vi "BestY for any element.vi"(7 "Element Position":dbl[](array[numeric]), 8 "error in (no error)":errorcluster, 9 "Enemys(T)\nAllys(F)":bool=TRUE, 10 "Game":refnum<class "Game.lvclass">, 11 "Utilities in":refnum<class "Utilities.lvclass">) -> (0 "error out":errorcluster, 2 "Goal Gap Normalizado(%do gol aberta)":dbl, 3 "Utilities out":refnum<class "Utilities.lvclass">)   [LabVIEW 2018, in "Utilities.lvclass"]
uses:
  Utilities.lvclass
  segment.ctl
  Game_class/Game.lvclass
  Game_class/Game.lvclass/Game.ctl
  Team_class/Team.lvclass/Team.ctl
  Object_class/Object.lvclass/Object.ctl
  Object_class/Read x.vi
  Object_class/Read y.vi
  <vilib>/Analysis/baseanly.llb/Real Dot Product.vi
  Game_class/Read FieldRef.vi
  Game_class/Read EnemyRef.vi
  Game_class/Read AllyRef.vi
  Team_class/Read RobotRef.vi
  Ally_class/Ally.lvclass
  Enemy_class/Enemy.lvclass
  Robot_class/Robot.lvclass
  Field_class/Field.lvclass
  <vilib>/Analysis/NI_AALBase.lvlib
panel:
  out "Vetor de gaps \ncorreto":T1[](array[typedef])
  out "Eclipse":bool
  out "Gap Coord":dbl[](array[numeric])
  out "Goal Gap":dbl
  out "Vetor de gaps":T1[](array[typedef])
  in  "Maior intervalo(T)\nMaior angulo(F)":bool
  in  "eclipse angle eps":dbl=0.035 format="%#_13g"
  out "Best y(for kick target)":dbl
  out "pilha output (merged)":T1[](array[typedef])
  out "Vetor de segmentos ordenado":T1[](array[typedef])
  out "Vetor de segmentos (sombras)":T1[](array[typedef])
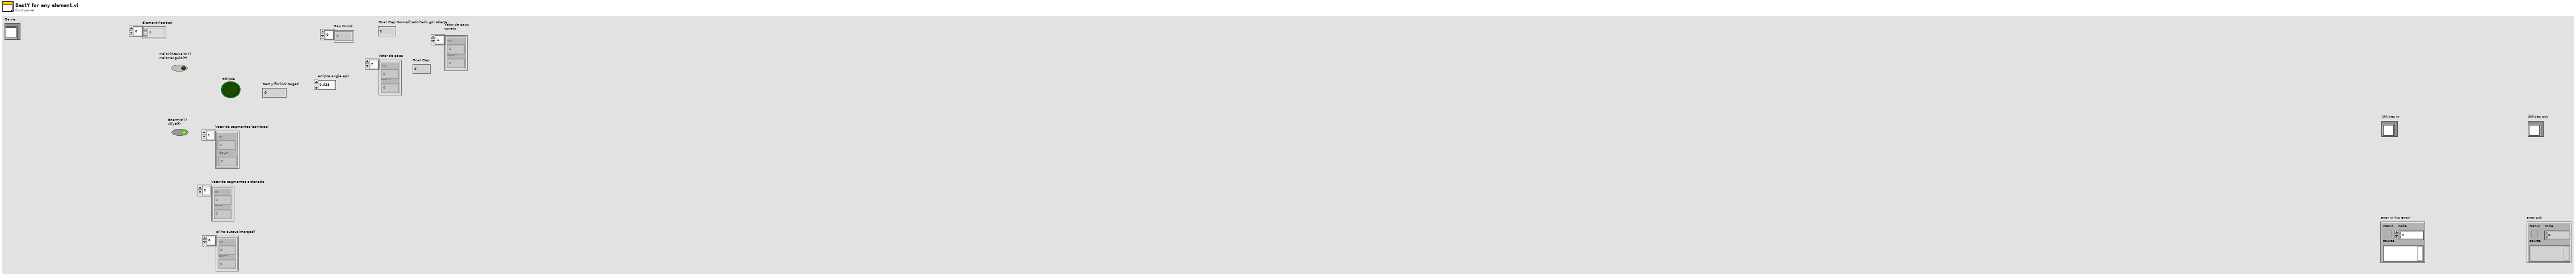
[diagram p1: front panel]
types:
  T1 = typedef "Utilities.lvclass/segment.ctl" = cluster{"up":dbl, "down":dbl}
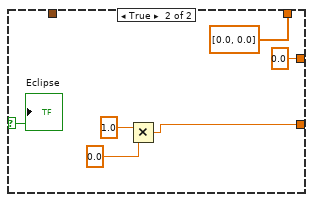
[diagram p4: hidden frame]
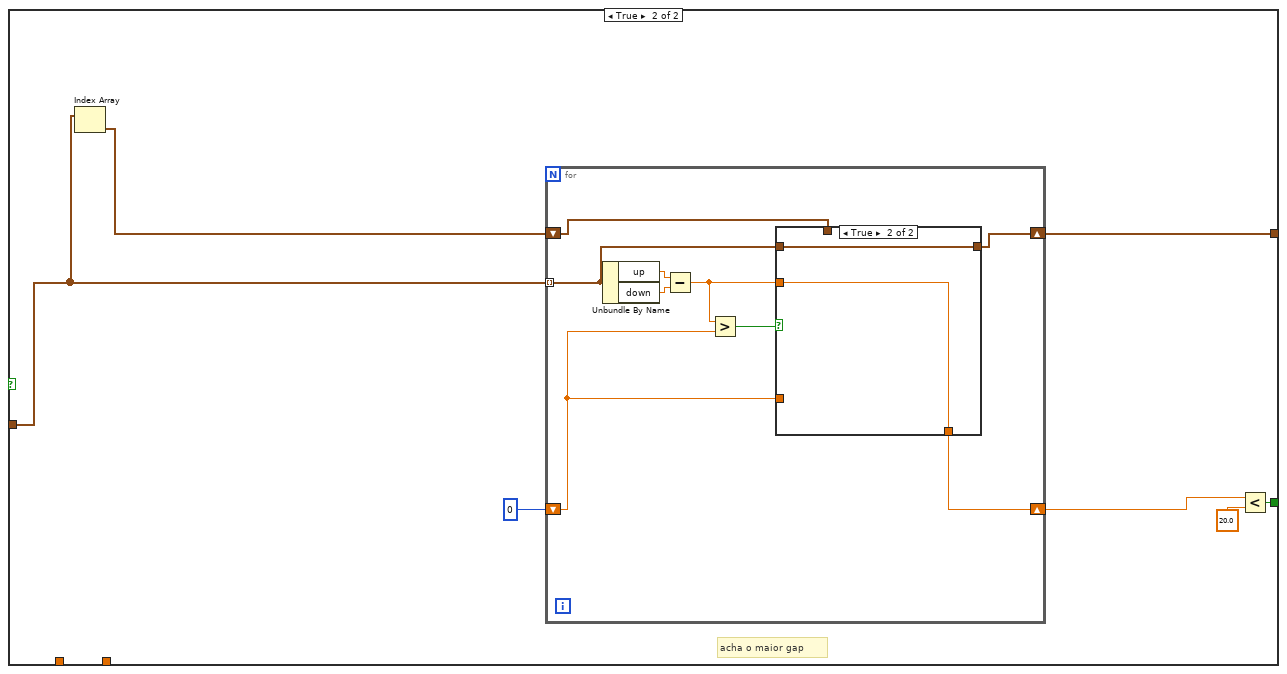
[diagram p6: hidden frame]
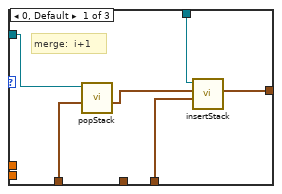
[diagram p8: hidden frame]
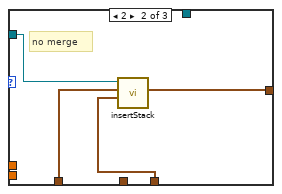
[diagram p9: hidden frame]
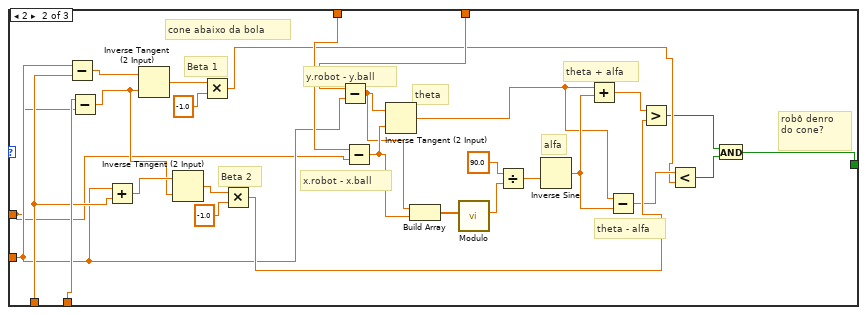
[diagram p11: hidden frame]
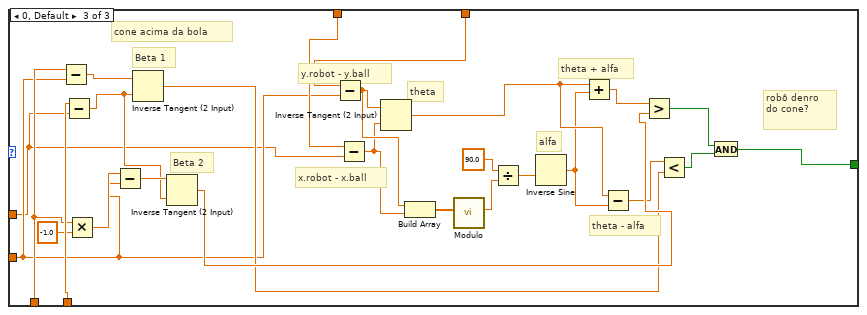
[diagram p12: hidden frame]
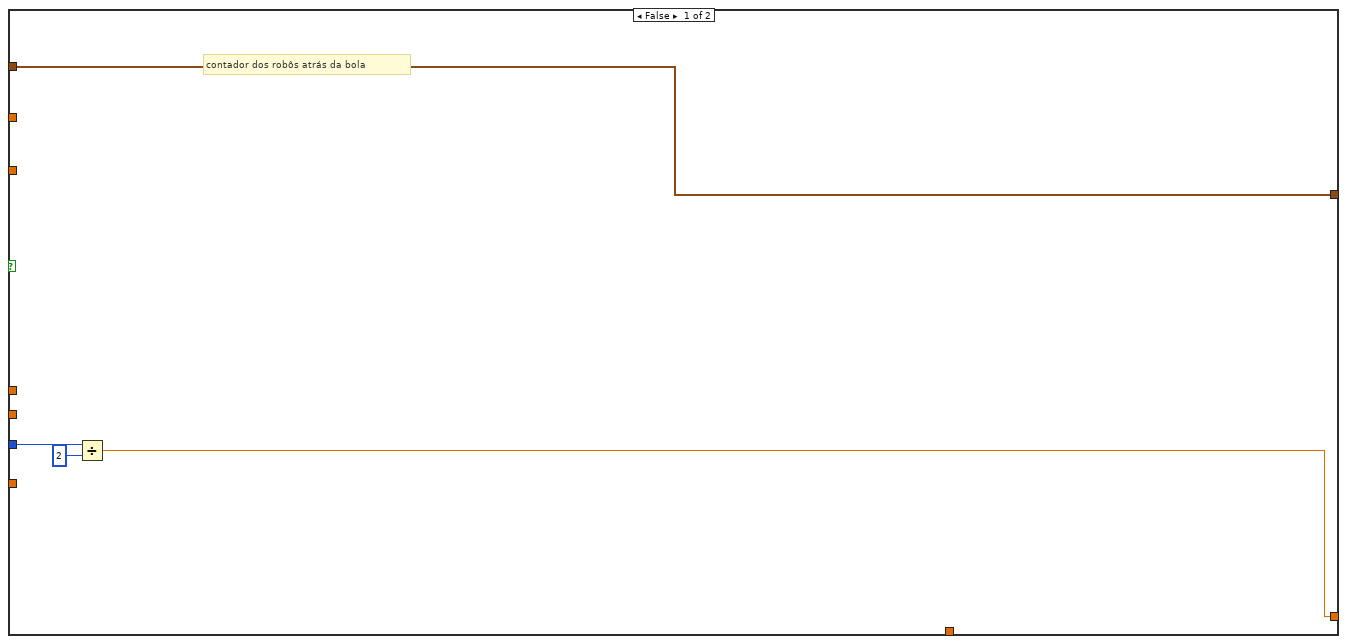
[diagram p13: hidden frame]
diagram:
  n1 = case shown="No Error" "error in (no error)" {
    selector: "error in (no error)" -> [w51 w398]
    tunnel: [w51 w398] -> w5
    tunnel: [w7 w397] -> w3
    tunnel: "Utilities in" -> [w7 w397]
    tunnel: "Game" -> [w9 _]
    tunnel: "Enemys(T)\nAllys(F)" -> [w8 _]
    frame No Error {
      # "default T"
      # "Default FALSE"
      # "goal_width/2"
      # "field_length/2"
      # "balls"
      # "vetor de gaps"
      # "upper"
      # "Wire the error cluster across even in the \"No Error\"\ncase so that warnings get propagated."
      n2 = property class="Game"(reference=w9) -> ("FieldRef"=w16:refnum<class "Field.lvclass">, "EnemyRef"=w13:refnum<class "Enemy.lvclass">, "AllyRef"=w12:refnum<class "Ally.lvclass">)  [unwired: 1 in, 2 out]
      n3 = property class="Enemy"(reference=w13) -> ("RobotRef"=w10:refnum<class "Robot.lvclass">[])  [unwired: 1 in, 2 out]
      n4 = property class="Ally"(reference=w12) -> ("RobotRef"=w11:refnum<class "Robot.lvclass">[])  [unwired: 1 in, 2 out]
      n5 = property class="Field"(reference=w16) -> ("field_length"=w15:i32, "field_width"=w14:i32)  [unwired: 1 in, 2 out]
      n6 = Select(t=w10, s=w8, f=w11) -> (s? t:f=w33:refnum<class "Robot.lvclass">[])
      n7 = Divide(x=w14, y=u32 2 ("x")) -> (x/y=w25:dbl)
      n8 = To Double Precision Float(number=w14) -> (double precision float=w17:dbl)
      n9 = for {
        shift-right: [w245] -> w36
        shift-left: T1[] [] -> [w244]
        tunnel: w15 -> [w223]
        tunnel: w25 -> [w225]
        tunnel: w25 -> [w242]
        shift-right: [w241] -> w34
        shift-left: _ -> [_]
        tunnel: w33 -> [w214] mode=indexing
        tunnel: w8 -> [w239]
        tunnel: "Element Position" -> [w217]
        # "y element"
        # "x element"
        # "y.robot"
        # "x.robot"
        # "field_length/2"
        # "goal_width/2"
        # "y element"
        # "x element"
        n10 = property class="Robot"(reference=w214) -> ("x"=w213:dbl, "y"=w212:dbl)  [unwired: 1 in, 2 out]
        n11 = Index Array(array=w217) -> (element #1=w216:dbl, element #2=w215:dbl)  [unwired: 2 in]
        n12 = Multiply(x=w213, y=-1.0) -> (x*y=w238:dbl)
        n13 = Absolute Value(x=w216) -> (abs(x)=w237:dbl)
        n14 = Absolute Value(x=w213) -> (abs(x)=w243:dbl)
        n15 = Select(t=w213, s=w239, f=w238) -> (s? t:f=w220:dbl)
        n16 = Greater?(x=w243, y=w237) -> (0:w218:bool)
        n17 = Multiply(x=w225, y=-1.0) -> (x*y=w229:dbl)
        n18 = Greater?(x=w215, y=w225) -> (0:w228:bool)
        n19 = Less?(x=w215, y=w229) -> (x < y?=w227:bool)
        n20 = Select(t=1, s=w228, f=0) -> (s? t:f=w235:i32)
        n21 = Select(t=0, s=w227, f=1) -> (s? t:f=w236:i32)
        n22 = Add(x=w235, y=w236) -> (x+y=w226:i32)
        n23 = Divide(x=w223, y=2.0) -> (x/y=w222:dbl)
        n24 = case shown="1" w226 {
          tunnel: w225 -> [w248 w274 w322]
          tunnel: w222 -> [w269 w294 w324]
          tunnel: w220 -> [w256 w281 w317]
          tunnel: w212 -> [w255 w282 w318]
          tunnel: [w257 w283 w308] -> w219
          tunnel: w216 -> [w246 w272 w300]
          tunnel: w215 -> [w247 w273 w301]
          frame 1 {
            # "robô denro\ndo cone?"
            # "cone centrado"
            # "theta - alfa"
            # "theta + alfa"
            # "theta"
            # "alfa"
            # "x.robot - x.element"
            # "y.robot - y.element"
            # "Beta 2"
            # "Beta 1"
            n25 = Subtract(x=w248, y=w247) -> (x-y=w270:dbl)
            n26 = Subtract(x=w269, y=w246) -> (x-y=w271:dbl)
            n27 = Add(x=w247, y=w248) -> (x+y=w268:dbl)
            n28 = Inverse Tangent (2 Input)(1:w271, 2:w270) -> (0:w251:dbl)
            n29 = Inverse Tangent (2 Input)(1:w271, 2:w268) -> (0:w267:dbl)
            n30 = Multiply(x=w267, y=-1.0) -> (x*y=w253:dbl)
            n31 = Subtract(x=w255, y=w247) -> (x-y=w258:dbl)
            n32 = Subtract(x=w256, y=w246) -> (x-y=w259:dbl)
            n33 = Inverse Tangent (2 Input)(1:w259, 2:w258) -> (0:w264:dbl)
            n34 = Build Array(w258, w259) -> (w260:dbl[])
            n35 = call "Modulo.vi"("2D vector"=w260) -> ("Modulo"=w261:dbl)  [unwired: 10 in]
            n36 = Divide(x=90.0, y=w261) -> (x/y=w262:dbl)
            n37 = Inverse Sine(1:w262) -> (0:w265:dbl)
            n38 = Add(x=w264, y=w265) -> (x+y=w254:dbl)
            n39 = Subtract(x=w264, y=w265) -> (x-y=w252:dbl)
            n40 = Greater?(x=w254, y=w253) -> (0:w249:bool)
            n41 = Less?(x=w252, y=w251) -> (x < y?=w250:bool)
            n42 = And(x=w249, y=w250) -> (x .and. y?=w257:bool)
          }
          frame 2 {
            # "robô denro\ndo cone?"
            # "cone abaixo da bola"
            # "theta - alfa"
            # "theta + alfa"
            # "theta"
            # "alfa"
            # "x.robot - x.ball"
            # "y.robot - y.ball"
            # "Beta 2"
            # "Beta 1"
            n43 = Subtract(x=w273, y=w274) -> (x-y=w296:dbl)
            n44 = Subtract(x=w294, y=w272) -> (x-y=w295:dbl)
            n45 = Add(x=w273, y=w274) -> (x+y=w297:dbl)
            n46 = Inverse Tangent (2 Input)(1:w295, 2:w296) -> (0:w292:dbl)
            n47 = Inverse Tangent (2 Input)(1:w295, 2:w297) -> (0:w298:dbl)
            n48 = Multiply(x=w292, y=-1.0) -> (x*y=w277:dbl)
            n49 = Multiply(x=w298, y=-1.0) -> (x*y=w279:dbl)
            n50 = Subtract(x=w282, y=w273) -> (x-y=w284:dbl)
            n51 = Subtract(x=w281, y=w272) -> (x-y=w285:dbl)
            n52 = Inverse Tangent (2 Input)(1:w285, 2:w284) -> (0:w290:dbl)
            n53 = Build Array(w284, w285) -> (w286:dbl[])
            n54 = call "Modulo.vi"("2D vector"=w286) -> ("Modulo"=w287:dbl)  [unwired: 10 in]
            n55 = Divide(x=90.0, y=w287) -> (x/y=w288:dbl)
            n56 = Inverse Sine(1:w288) -> (0:w291:dbl)
            n57 = Add(x=w290, y=w291) -> (x+y=w280:dbl)
            n58 = Subtract(x=w290, y=w291) -> (x-y=w278:dbl)
            n59 = Greater?(x=w280, y=w279) -> (0:w275:bool)
            n60 = Less?(x=w278, y=w277) -> (x < y?=w276:bool)
            n61 = And(x=w275, y=w276) -> (x .and. y?=w283:bool)
          }
          frame 0, Default {
            # "robô denro\ndo cone?"
            # "cone acima da bola"
            # "theta - alfa"
            # "theta + alfa"
            # "theta"
            # "alfa"
            # "x.robot - x.ball"
            # "y.robot - y.ball"
            # "Beta 2"
            # "Beta 1"
            n62 = Subtract(x=w322, y=w301) -> (x-y=w325:dbl)
            n63 = Subtract(x=w324, y=w300) -> (x-y=w319:dbl)
            n64 = Multiply(x=w322, y=-1.0) -> (x*y=w321:dbl)
            n65 = Subtract(x=w321, y=w301) -> (x-y=w320:dbl)
            n66 = Inverse Tangent (2 Input)(1:w319, 2:w325) -> (0:w303:dbl)
            n67 = Inverse Tangent (2 Input)(1:w319, 2:w320) -> (0:w306:dbl)
            n68 = Subtract(x=w318, y=w301) -> (x-y=w316:dbl)
            n69 = Subtract(x=w317, y=w300) -> (x-y=w315:dbl)
            n70 = Inverse Tangent (2 Input)(1:w315, 2:w316) -> (0:w310:dbl)
            n71 = Build Array(w316, w315) -> (w314:dbl[])
            n72 = call "Modulo.vi"("2D vector"=w314) -> ("Modulo"=w313:dbl)  [unwired: 10 in]
            n73 = Divide(x=90.0, y=w313) -> (x/y=w312:dbl)
            n74 = Inverse Sine(1:w312) -> (0:w309:dbl)
            n75 = Add(x=w310, y=w309) -> (x+y=w307:dbl)
            n76 = Subtract(x=w310, y=w309) -> (x-y=w304:dbl)
            n77 = Greater?(x=w307, y=w306) -> (0:w305:bool)
            n78 = Less?(x=w304, y=w303) -> (x < y?=w302:bool)
            n79 = And(x=w305, y=w302) -> (x .and. y?=w308:bool)
          }
        }
        n80 = And(x=w218, y=w219) -> (x .and. y?=w221:bool)
        n81 = case shown="True" w221 {
          tunnel: [w329 w336] -> w245
          tunnel: w244 -> [w329 w338]
          tunnel: w223 -> [w328 w343]
          tunnel: w225 -> [_ w342]
          tunnel: w242 -> [_ w335]
          tunnel: [w326 w334] -> w241
          tunnel: w212 -> [_ w333]
          tunnel: w220 -> [_ w332]
          tunnel: w216 -> [_ w330]
          tunnel: w215 -> [_ w331]
          frame False {
            # "contador dos robôs atrás da bola"
            n82 = Divide(x=w328, y=u32 2) -> (x/y=w326:dbl)
          }
          frame True {
            n83 = flat-sequence {
              tunnel: w333 -> [w378]
              tunnel: w343 -> [w374]
              tunnel: w342 -> [w359]
              tunnel: [w349] -> w341
              tunnel: [w348] -> w340
              tunnel: [w360] -> w339
              tunnel: w338 -> [w353]
              tunnel: [w353] -> w337
              tunnel: [w347] -> w334
              tunnel: w332 -> [w346]
              tunnel: w331 -> [w344]
              tunnel: w330 -> [w345]
              tunnel: w341 -> [w382]
              tunnel: w340 -> [w381]
              tunnel: w339 -> [w383]
              tunnel: w337 -> [w384]
              tunnel: [w380] -> w336
              tunnel: w335 -> [w379]
              frame #0 {
                # "theta - alfa"
                # "alfa + theta"
                # "theta"
                # "alfa"
                # "x.robot - x.element"
                # "y.robot - y.element"
                n84 = Divide(x=w374, y=u32 2 ("x")) -> (x/y=w347:dbl)
                n85 = Subtract(x=w346, y=w345) -> (x-y=w357:dbl)
                n86 = Subtract(x=w378, y=w344) -> (x-y=w358:dbl)
                n87 = Multiply(x=w359, y=-1.0) -> (x*y=w365:dbl)
                n88 = Subtract(x=w347, y=w345) -> (x-y=w350:dbl)
                n89 = Inverse Tangent (2 Input)(1:w357, 2:w358) -> (0:w356:dbl)
                n90 = Build Array(w358, w357) -> (w377:dbl[])
                n91 = call "Modulo.vi"("2D vector"=w377) -> ("Modulo"=w375:dbl)  [unwired: 10 in]
                n92 = Divide(x=90.0, y=w375) -> (x/y=w355:dbl)
                n93 = Inverse Sine(1:w355) -> (0:w354:dbl)
                n94 = Subtract(x=w356, y=w354) -> (x-y=w370:dbl)
                n95 = Tangent(1:w370) -> (0:w369:dbl)
                n96 = Add(x=w356, y=w354) -> (x+y=w372:dbl)
                n97 = Tangent(1:w372) -> (0:w371:dbl)
                n98 = Multiply(x=w369, y=w350) -> (x*y=w351:dbl)
                n99 = Multiply(x=w371, y=w350) -> (x*y=w352:dbl)
                n100 = Add(x=w351, y=w344) -> (x+y=w348:dbl)
                n101 = Add(x=w352, y=w344) -> (x+y=w349:dbl)
                n102 = Less?(x=w349, y=w365) -> (x < y?=w364:bool)
                n103 = Less?(x=w348, y=w365) -> (x < y?=w363:bool)
                n104 = Greater?(x=w348, y=w359) -> (0:w367:bool)
                n105 = Greater?(x=w349, y=w359) -> (0:w368:bool)
                n106 = And(x=w368, y=w367) -> (x .and. y?=w362:bool)
                n107 = And(x=w364, y=w363) -> (x .and. y?=w361:bool)
                n108 = Or(x=w362, y=w361) -> (x .or. y?=w360:bool)
              }
              frame #1 {
                # "goal_width/2"
                n109 = case shown="False" w383 {
                  tunnel: [w393 w396] -> w380
                  tunnel: w384 -> [w392 w396]
                  tunnel: w382 -> [w391 _]
                  tunnel: w381 -> [w389 _]
                  tunnel: w379 -> [w388 _]
                  frame False {
                    n110 = Max & Min(x=w391, y=w388) -> (min(x,y)=w390:dbl)  [unwired: 1 out]
                    n111 = Multiply(x=w388, y=-1.0) -> (x*y=w386:dbl)
                    n112 = Max & Min(x=w389, y=w386) -> (max(x,y)=w385:dbl)  [unwired: 1 out]
                    n113 = Bundle(cluster=T1 {"up"=0.0, "down"=0.0} ("segment 2"), "up"=w390, "down"=w385) -> (w394:T1)
                    n114 = Insert Into Array(array=w392, new element=w394) -> (w393:T1[])  [unwired: 1 in]
                  }
                  frame True {
                  }
                }
              }
            }
          }
        }
      }
      "Vetor de segmentos (sombras)" <- w36
      n115 = Sort 1D Array(array=w36) -> (sorted array=w48:T1[])
      "Vetor de segmentos ordenado" <- w48
      n116 = Index Array(array=w48) -> (element=w47:T1)  [unwired: 1 in]
      n117 = call-dynamic "insertStack.vi"("novo elemento"=w47, "pilha input"=T1[] [], "Utilities in"=w7) -> ("pilha output"=w45:T1[])  [unwired: 5 in, 2 out]
      n118 = for {
        shift-right: [w171] -> w44
        shift-left: w45 -> [w173]
        tunnel: w48 -> [w172] mode=indexing
        i -> [w174]
        n119 = case shown="Default" w174 {
          tunnel: w173 -> [w179 w211]
          tunnel: w172 -> [w182 _]
          tunnel: [w180 w211] -> w171
          frame Default {
            w175 = refnum<class "Utilities.lvclass"> refnum ("Utilities in")
            # "pilha"
            # "i+1"
            # "i"
            # "i+1"
            # "i"
            n120 = call-dynamic "topStack.vi"("pilha input"=w179, "Utilities in"=w175) -> ("top"=w181:T1)  [unwired: 7 in, 2 out]
            n121 = Unbundle By Name(w181) -> ("up"=w178:dbl, "down"=w183:dbl)
            n122 = Unbundle By Name(w182) -> ("down"=w177:dbl, "up"=w184:dbl)
            n123 = Greater Or Equal?(x=w177, y=w178) -> (x >= y?=w176:bool)
            n124 = Less?(x=w177, y=w183) -> (x < y?=w186:bool)
            n125 = Select(t=1, s=w176, f=0) -> (s? t:f=w188:i32)
            n126 = Select(t=0, s=w186, f=1) -> (s? t:f=w187:i32)
            n127 = Add(x=w188, y=w187) -> (x+y=w185:i32)
            n128 = case shown="1" w185 {
              tunnel: w184 -> [_ _ w209]
              tunnel: w183 -> [_ _ w208]
              tunnel: w181 -> [_ _ _]
              tunnel: w182 -> [w195 w201 _]
              tunnel: [w198 w200 w204] -> w180
              tunnel: w179 -> [w197 w202 w207]
              tunnel: w175 -> [w194 _ _]
              tunnel: w175 -> [w193 w199 w203]
              frame 0, Default {
                # "merge:  i+1"
                n129 = call-dynamic "popStack.vi"("pilha input"=w197, "Utilities in"=w193) -> ("pilha output"=w196:T1[])  [unwired: 7 in, 2 out]
                n130 = call-dynamic "insertStack.vi"("novo elemento"=w195, "pilha input"=w196, "Utilities in"=w194) -> ("pilha output"=w198:T1[])  [unwired: 5 in, 2 out]
              }
              frame 2 {
                # "no merge"
                n131 = call-dynamic "insertStack.vi"("novo elemento"=w201, "pilha input"=w202, "Utilities in"=w199) -> ("pilha output"=w200:T1[])  [unwired: 5 in, 2 out]
              }
              frame 1 {
                # "merge top i+1 down i"
                n132 = Bundle(cluster=T1 {"up"=0.0, "down"=0.0} ("segment 2"), "up"=w209, "down"=w208) -> (w205:T1)
                n133 = call-dynamic "popStack.vi"("pilha input"=w207, "Utilities in"=w203) -> ("pilha output"=w206:T1[])  [unwired: 7 in, 2 out]
                n134 = call-dynamic "insertStack.vi"("novo elemento"=w205, "pilha input"=w206, "Utilities in"=w203) -> ("pilha output"=w204:T1[])  [unwired: 5 in, 2 out]
              }
            }
          }
          frame 0 {
          }
        }
      }
      "pilha output (merged)" <- w44
      n135 = Reverse 1D Array(array=w44) -> (reversed array=w43:T1[])
      n136 = for {
        tunnel: w43 -> [w170] mode=indexing
        shift-right: [w164] -> w40
        shift-left: T1[] [] -> [w166]
        shift-right: [w165] -> w39
        shift-left: w25 -> [w167]
        n137 = Unbundle By Name(w170) -> ("up"=w163:dbl, "down"=w165:dbl)
        n138 = Bundle(cluster=T1 {"up"=0.0, "down"=0.0} ("segment 2"), "up"=w167, "down"=w163) -> (w169:T1)
        n139 = Insert Into Array(array=w166, new element=w169) -> (w164:T1[])  [unwired: 1 in]
      }
      n140 = Multiply(x=w25, y=-1.0) -> (x*y=w37:dbl)
      n141 = Bundle(cluster=T1 {"up"=0.0, "down"=0.0} ("segment 2"), "up"=w39, "down"=w37) -> (w42:T1)
      n142 = Insert Into Array(array=w40, new element=w42) -> (w26:T1[])  [unwired: 1 in]
      n143 = Array Size(array=w26) -> (size(s)=w28:i32)
      n144 = Decrement(x=w28) -> (x-1=w27:i32)
      n145 = for {
        N: w27 -> [_]
        shift-right: [w70] -> w24
        shift-left: w26 -> [w72]
        i -> [w71]
        n146 = Increment(x=w71) -> (x+1=w80:i32)
        n147 = Index Array(array=w72, index=w71) -> (element=w73:T1)
        n148 = Index Array(array=w72, index=w80) -> (element=w79:T1)
        n149 = Unbundle By Name(w79) -> ("up"=w77:dbl, "down"=w74:dbl)
        n150 = Unbundle By Name(w73) -> ("up"=w75:dbl, "down"=w78:dbl)
        n151 = Equal?(x=w78, y=w77) -> (x = y?=w76:bool)
        n152 = case shown="True" w76 {
          tunnel: w75 -> [_ w90]
          tunnel: w74 -> [_ w89]
          tunnel: w73 -> [_ w88]
          tunnel: w72 -> [w81 w86]
          tunnel: w71 -> [_ w83]
          tunnel: [w81 w82] -> w70
          frame False {
          }
          frame True {
            n153 = Bundle By Name(cluster=w88, "up"=w90, "down"=w89) -> (w84:T1)
            n154 = Delete From Array(array=w86, length=2, index=w83) -> (array with subset deleted=w85:T1[])  [unwired: 1 out]
            n155 = Insert Into Array(array=w85, index=w83, new element=w84) -> (w82:T1[])
          }
        }
      }
      "Vetor de gaps" <- w24
      n156 = for {
        tunnel: w25 -> [w61]
        tunnel: w24 -> [w54] mode=indexing
        shift-right: [w56] -> w21
        shift-left: T1[] [] -> [w55]
        n157 = Unbundle By Name(w54) -> ("up"=w53:dbl, "down"=w52:dbl)
        n158 = Multiply(x=w61, y=-1.0) -> (x*y=w60:dbl)
        n159 = Greater?(x=w53, y=w61) -> (0:w58:bool)
        n160 = Less?(x=w52, y=w60) -> (x < y?=w57:bool)
        n161 = Or(x=w58, y=w57) -> (x .or. y?=w59:bool)
        n162 = case shown="False" w59 {
          tunnel: [w63 w66] -> w56
          tunnel: w55 -> [w63 w67]
          tunnel: w53 -> [_ w64]
          tunnel: w52 -> [_ w65]
          frame True {
          }
          frame False {
            n163 = Bundle(cluster=T1 {"up"=0.0, "down"=0.0} ("segment 2"), "up"=w64, "down"=w65) -> (w68:T1)
            n164 = Insert Into Array(array=w67, new element=w68) -> (w66:T1[])  [unwired: 1 in]
          }
        }
      }
      "Vetor de gaps \ncorreto" <- w21
      n165 = case shown="False" "Maior intervalo(T)\nMaior angulo(F)" {
        tunnel: [w110 w146] -> w31
        tunnel: [w109 w144] -> w32
        tunnel: w21 -> [w114 w145]
        tunnel: w34 -> [w113 _]
        tunnel: "Element Position" -> [w108 _]
        frame False {
          # "acha o maior ângulo"
          n166 = Index Array(array=w108) -> (element #1=w107:dbl, element #2=w106:dbl)  [unwired: 2 in]
          n167 = Index Array(array=w114) -> (element=w115:T1)  [unwired: 1 in]
          n168 = for {
            tunnel: w114 -> [w136] mode=indexing
            shift-right: [w137] -> w112
            shift-left: 0 -> [w119]
            shift-right: [w135] -> w109
            shift-left: w115 -> [w134]
            tunnel: w107 -> [w118]
            tunnel: w106 -> [w117]
            tunnel: w113 -> [w133]
            # "theta"
            # "cos (theta)"
            # "vetor bola-down"
            # "vetor bola-up"
            n169 = Unbundle By Name(w136) -> ("up"=w132:dbl, "down"=w129:dbl)
            n170 = Subtract(x=w133, y=w118) -> (x-y=w130:dbl)
            n171 = Subtract(x=w129, y=w117) -> (x-y=w128:dbl)
            n172 = Subtract(x=w132, y=w117) -> (x-y=w131:dbl)
            n173 = Build Array(w130, w128) -> (w126:dbl[])
            n174 = Build Array(w130, w131) -> (w127:dbl[])
            n175 = call-poly <vilib>:"Dot Product.vi"("Y Vector"=w126, "X Vector"=w127) -> ("X * Y"=w123:dbl)  [unwired: 1 out]
            n176 = call "Modulo.vi"("2D vector"=w127) -> ("Modulo"=w125:dbl)  [unwired: 10 in]
            n177 = call "Modulo.vi"("2D vector"=w126) -> ("Modulo"=w124:dbl)  [unwired: 10 in]
            n178 = Multiply(x=w125, y=w124) -> (x*y=w122:dbl)
            n179 = Divide(x=w123, y=w122) -> (x/y=w121:dbl)
            n180 = Inverse Cosine(1:w121) -> (0:w120:dbl)
            n181 = Greater?(x=w120, y=w119) -> (0:w138:bool)
            n182 = case shown="True" w138 {
              tunnel: w120 -> [_ w142]
              tunnel: [w139 w142] -> w137
              tunnel: w136 -> [_ w141]
              tunnel: [w140 w141] -> w135
              tunnel: w134 -> [w140 _]
              tunnel: w119 -> [w139 _]
              frame False {
              }
              frame True {
              }
            }
          }
          n183 = Less?(x=w112, y="eclipse angle eps") -> (x < y?=w110:bool)
        }
        frame True {
          # "acha o maior gap"
          n184 = Index Array(array=w145) -> (element=w148:T1)  [unwired: 1 in]
          n185 = for {
            tunnel: w145 -> [w153] mode=indexing
            shift-right: [w154] -> w147
            shift-left: 0 -> [w151]
            shift-right: [w152] -> w144
            shift-left: w148 -> [w150]
            n186 = Unbundle By Name(w153) -> ("up"=w158:dbl, "down"=w157:dbl)
            n187 = Subtract(x=w158, y=w157) -> (x-y=w155:dbl)
            n188 = Greater?(x=w155, y=w151) -> (0:w156:bool)
            n189 = case shown="True" w156 {
              tunnel: w155 -> [_ w162]
              tunnel: [w160 w162] -> w154
              tunnel: w153 -> [_ w161]
              tunnel: [w159 w161] -> w152
              tunnel: w151 -> [w160 _]
              tunnel: w150 -> [w159 _]
              frame False {
              }
              frame True {
              }
            }
          }
          n190 = Less?(x=w147, y=20.0) -> (x < y?=w146:bool)
        }
      }
      n191 = case shown="False" w31 {
        selector: w31 -> [_ w105]
        tunnel: w32 -> [w97 _]
        tunnel: [w96 w102] -> w29
        tunnel: [w94 0.0] -> w18
        tunnel: [w91 dbl[] [0.0, 0.0] ("Gap Coord")] -> w30
        frame False {
          n192 = Unbundle By Name(w97) -> ("up"=w93:dbl, "down"=w92:dbl)
          n193 = Subtract(x=w93, y=w92) -> (x-y=w95:dbl)
          n194 = Build Array(w93, w92) -> (w91:dbl[])
          n195 = Add(x=w93, y=w92) -> (x+y=w98:dbl)
          n196 = Absolute Value(x=w95) -> (abs(x)=w94:dbl)
          n197 = Divide(x=w98, y=2.0) -> (x/y=w96:dbl)
        }
        frame True {
          n198 = Multiply(x=1.0, y=0.0) -> (x*y=w102:dbl)
          "Eclipse" <- w105
        }
      }
      "Best y(for kick target)" <- w29
      "Goal Gap" <- w18
      "Gap Coord" <- w30
      n199 = Divide(x=w18, y=w17) -> (x/y=→"Goal Gap Normalizado(%do gol aberta)":dbl)
    }
    frame Error {
    }
  }
  "error out" <- w5
  "Utilities out" <- w3
